vi "MPExxx_set_modulation_information.vi"(2 "error in (no error)":errorcluster, 3 "Modulation Type":u16(ring) items=["Multiplication", "Addition"], 4 "Select Output to Modulate":i8(ring) items=["None", "Voltage", "Current"], 5 "VISA session":refnum<visa-resource-name>) -> (0 "error out":errorcluster, 1 "dup VISA session":refnum<visa-resource-name>)   [LabVIEW 2012]
doc: "This VI form sets the mode of modulation and modulation type."
uses:
  MPExxx Globals.gbl
panel:
  # "MAGNA-POWER"
  # "Electronics"
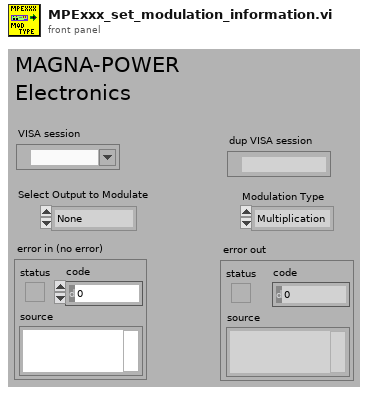
[diagram p1: front panel]
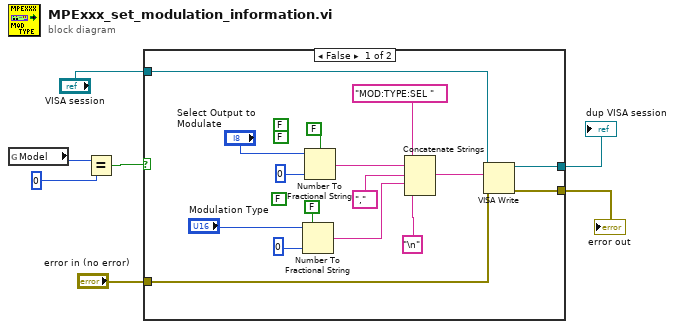
[diagram p0: block diagram]
diagram:
  n1 = global read "MPExxx Globals.gbl" "Model"() -> (w5:u8)
  n2 = Equal?(x=w5, y=0) -> (x = y?=w7:bool)
  n3 = case shown="False" w7 {
    tunnel: "VISA session" -> [w11 w25]
    tunnel: "error in (no error)" -> [w10 w24]
    tunnel: [w9 w24] -> w2
    tunnel: [w8 w25] -> w1
    frame False {
      (unwired) FALSE ("use system decimal point (T)")
      (unwired) FALSE ("use system decimal point (T)")
      (unwired) FALSE ("use system decimal point (T)")
      (unwired) FALSE ("use system decimal point (T)")
      n4 = Number To Fractional String(use system decimal point (T)=FALSE, number="Modulation Type", precision (6)=0) -> (F-format string=w14:string)  [unwired: 1 in]
      n5 = Number To Fractional String(use system decimal point (T)=FALSE, number="Select Output to Modulate", precision (6)=0) -> (F-format string=w16:string)  [unwired: 1 in]
      n6 = Concatenate Strings("MOD:TYPE:SEL ", w16, ",", w14, "\n") -> (w22:string)
      n7 = VISA Write(VISA resource name=w11, write buffer=w22, error in (no error)=w10) -> (VISA resource name out=w8:refnum<visa-resource-name>, error out=w9:errorcluster)  [unwired: 1 out]
    }
    frame True {
    }
  }
  "error out" <- w2
  "dup VISA session" <- w1
